vi "test.copy.vi"(8 "error in (no error)":errorcluster, 11 "TestCase in":refnum<class "TestCase.Pointer.lvclass">) -> (0 "error out":errorcluster, 3 "TestCase out":refnum<class "TestCase.Pointer.lvclass">)   [LabVIEW 2016, in "TestCase.Pointer.lvclass"]
uses:
  TestCase.Pointer.lvclass
  pointer methods.ctl
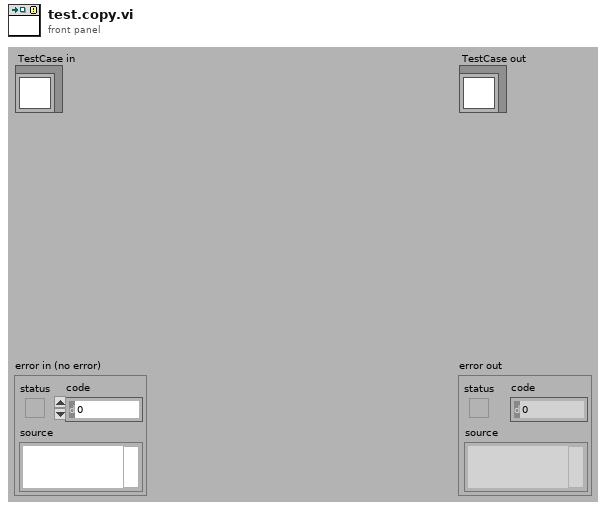
[diagram p1: front panel]
types:
  T1 = typedef "TestCase.Pointer.lvclass/pointer methods.ctl" = enum16{"Advanced Copy", "Check If Equal Size", "Check If Equal Contents", "Check", "Clear Subset", "Clear", "Copy All", "Copy", "Duplicate", "Read", "Swap", "Write"}
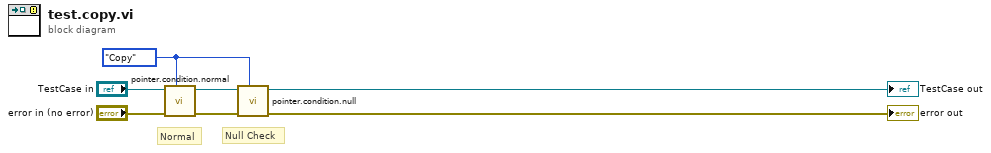
[diagram p0: block diagram]
diagram:
  w3 = pointer_methods."Copy" ("Pointer methods")
  # "Null Check"
  # "Normal"
  n1 = call "pointer.condition.normal.vi"("Pointer methods"=w3, "error in (no error)"="error in (no error)", "TestCase in"="TestCase in") -> ("error out"=w4:errorcluster, "TestCase out"=w5:refnum<class "TestCase.Pointer.lvclass">)  [unwired: 7 in]
  n2 = call "pointer.condition.null.vi"("Pointer methods"=w3, "error in (no error)"=w4, "TestCase in"=w5) -> ("error out"=→"error out":errorcluster, "TestCase out"=→"TestCase out":refnum<class "TestCase.Pointer.lvclass">)  [unwired: 7 in]
